vi "Microfone3.vi"() -> ()   [LabVIEW 2014]
uses:
  <vilib>/myRIO/Instrument Drivers/Onboard IO/AI/typedefs/AI Reference.ctl
  <vilib>/myRIO/Common/Instrument Driver Framework/Utilities/typedefs/myRIO Generic Hardware Reference.ctl
  <vilib>/myRIO/Common/Instrument Driver Framework/Utilities/typedefs/Hardware Version Enum.ctl
  <vilib>/myRIO/Common/Instrument Driver Framework/Utilities/typedefs/myRIO v1.0 Reference.ctl
  <vilib>/myRIO/Common/Instrument Driver Framework/Utilities/typedefs/Generic FPGA Reference.ctl
  <vilib>/myRIO/Common/Instrument Driver Framework/myRIO v1.0/AI/typedefs/AI Channels List.ctl
  <vilib>/myRIO/Common/Instrument Driver Framework/myRIO v1.0/AI/typedefs/AI Channels Enum.ctl
  <vilib>/myRIO/Common/Instrument Driver Framework/Utilities/typedefs/Analog Scaling Constants List.ctl
  <vilib>/myRIO/Common/Instrument Driver Framework/Utilities/typedefs/Analog Scaling Constants.ctl
  <vilib>/userdefined/High Color/nirio_resource_hc.ctl
  <vilib>/myRIO/Common/Instrument Driver Framework/Utilities/vis/Is FPGA Ref Available.vi
  <vilib>/myRIO/Common/Instrument Driver Framework/myRIO v1.0/AI/vis/myRIO v1.1 Open AI.vi
  <vilib>/myRIO/Instrument Drivers/Onboard IO/AI/vis/Read.vi
  <vilib>/myRIO/Common/Instrument Driver Framework/Utilities/vis/Validate Channels.vi
  <vilib>/myRIO/Common/Instrument Driver Framework/myRIO v1.0/AI/vis/myRIO v1.0 Reserve AI.vi
  <vilib>/myRIO/Common/Instrument Driver Framework/myRIO v1.0/AI/vis/myRIO v1.0 Build MUX Configuration AI.vi
  <vilib>/myRIO/Common/Instrument Driver Framework/myRIO v1.0/Resource Manager/vis/myRIO v1.0 Reserve Channel List.vi
  <vilib>/myRIO/Common/Instrument Driver Framework/myRIO v1.0/Resource Manager/vis/myRIO v1.0 Reserve Channel.vi
  <vilib>/myRIO/Common/Instrument Driver Framework/myRIO v1.0/Resource Manager/vis/myRIO v1.0 Unreserve Channel.vi
  <vilib>/myRIO/Common/Instrument Driver Framework/myRIO v1.0/Resource Manager/vis/myRIO v1.0 Build Mutex Name.vi
  <vilib>/Utility/VariantDataType/GetNumericInfo.vi
  <vilib>/Utility/error.llb/Error Cluster From Error Code.vi
  <vilib>/myRIO/Common/Instrument Driver Framework/myRIO v1.0/myRIO v1.1 Open.vi
  <vilib>/myRIO/Common/Instrument Driver Framework/myRIO v1.0/AI/vis/myRIO v1.0 Get Scaling Constants AI.vi
  <vilib>/myRIO/Common/Instrument Driver Framework/Utilities/vis/IO Manager.vi
  <vilib>/myRIO/Common/Instrument Driver Framework/Utilities/vis/Configuration Manager.vi
  <vilib>/myRIO/Common/Instrument Driver Framework/myRIO v1.0/myRIO v1.0 Close.vi
  <vilib>/myRIO/Common/Instrument Driver Framework/myRIO v1.0/AI/vis/myRIO v1.0 Read AI.vi
  <vilib>/measure/matone.llb/Extract Multiple Tone Information N Chan.vi
  <vilib>/express/express analysis/Spectral/Block/exnSpectralBlock spectral measurements RMS poly.vi
  <vilib>/express/express analysis/Spectral/Block/exnSpectralBlock spectral measurements RMS DDT.vi
  <vilib>/myRIO/Express VI/Onboard IO/AI/AI Express VI.xnode
  <vilib>/myRIO/Instrument Drivers/Onboard IO/AI/vis/myRIO AI Open.xnode
  <vilib>/express/express analysis/Spectral/XNode/ExpressSpectralMeasurementsBlockNode.xnode
  <vilib>/measure/NI_MAPro.lvlib
  <vilib>/gmath/NI_Gmath.lvlib
  <vilib>/myRIO/Instrument Drivers/Onboard IO/AI/AI.lvlib
panel:
  out "size(s) 2":i32
  out "size(s)":i32
  out "XY Graph":cluster{"xi used":dbl[], "yi":dbl[]}(graph)
  in  "Threshold":dbl=0.001 format="%#_6p"
  out "Primeira amplitude":dbl
  out "Primeira frequência":dbl
  out "multiple tone information":T1(array[cluster]) {"multiple tone information"."detected phase (deg)" format="%_6g"; "multiple tone information"."detected amplitude" format="%_6p"; "multiple tone information"."detected frequency" format="%_6p"}
  in  "Stop Button":bool
  out "Espectro de Amplitudes":dynamicdata(graph)
  out "Waveform Graph":dynamicdata(graph)
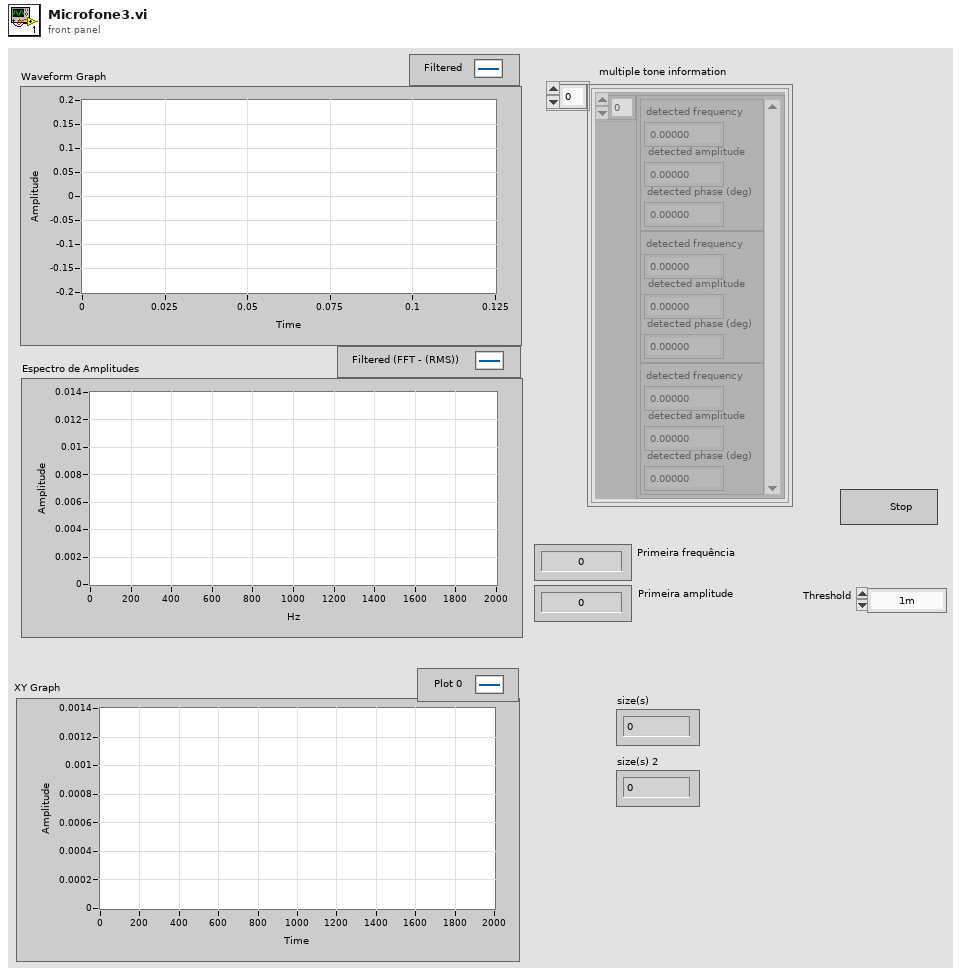
[diagram p1: front panel]
types:
  T1 = cluster{"multiple tone information":cluster{"detected frequency":dbl, "detected amplitude":dbl, "detected phase (deg)":dbl}[]}[]
  T2 = cluster{"averaging mode":u16, "weighting mode":u16, "number of averages":u32}
  T3 = cluster{"dB On (F)":bool, "unwrap phase (F)":bool, "convert to degree (F)":bool}
  T4 = typedef "AI.lvlib/AI Reference.ctl" = cluster{"myRIO Reference":T5, "AI Channels List":T9, "AI Scaling Constants List":T11}
  T5 = typedef "myRIO Generic Hardware Reference.ctl" = cluster{"myRIO Model":T6, "myRIO Hardware Reference":T7}
  T6 = typedef "Hardware Version Enum.ctl" = enum16{"Unknown", "myRIO-1900", "myRIO-1950"}
  T7 = typedef "myRIO v1.0 Reference.ctl" = cluster{"Generic FPGA Reference":T8, "Allow multiple opens":bool}
  T8 = typedef "Generic FPGA Reference.ctl" = refnum<k20>
  T9 = typedef "AI Channels List.ctl" = T10[]
  T10 = typedef "AI Channels Enum.ctl" = enum16{"Not Connected", "AudioIn/Left", "AudioIn/Right", "C/AI0", "C/AI1", "A/AI0", "A/AI1", "A/AI2", "A/AI3", "B/AI0", "B/AI1", "B/AI2", "B/AI3"}
  T11 = typedef "Analog Scaling Constants List.ctl" = T12[]
  T12 = typedef "Analog Scaling Constants.ctl" = cluster{"LSB Weight (Volts)":dbl, "Offset (Volts)":dbl, "Signed?":bool}
  T13 = typedef "nirio_resource_hc.ctl" = tag
  T14 = cluster{"multiple tone information":cluster{"detected frequency":dbl, "detected amplitude":dbl, "detected phase (deg)":dbl}[]}
  T15 = cluster{"detected frequency":dbl, "detected amplitude":dbl, "detected phase (deg)":dbl}[]
  T16 = cluster{"detected frequency":dbl, "detected amplitude":dbl, "detected phase (deg)":dbl}
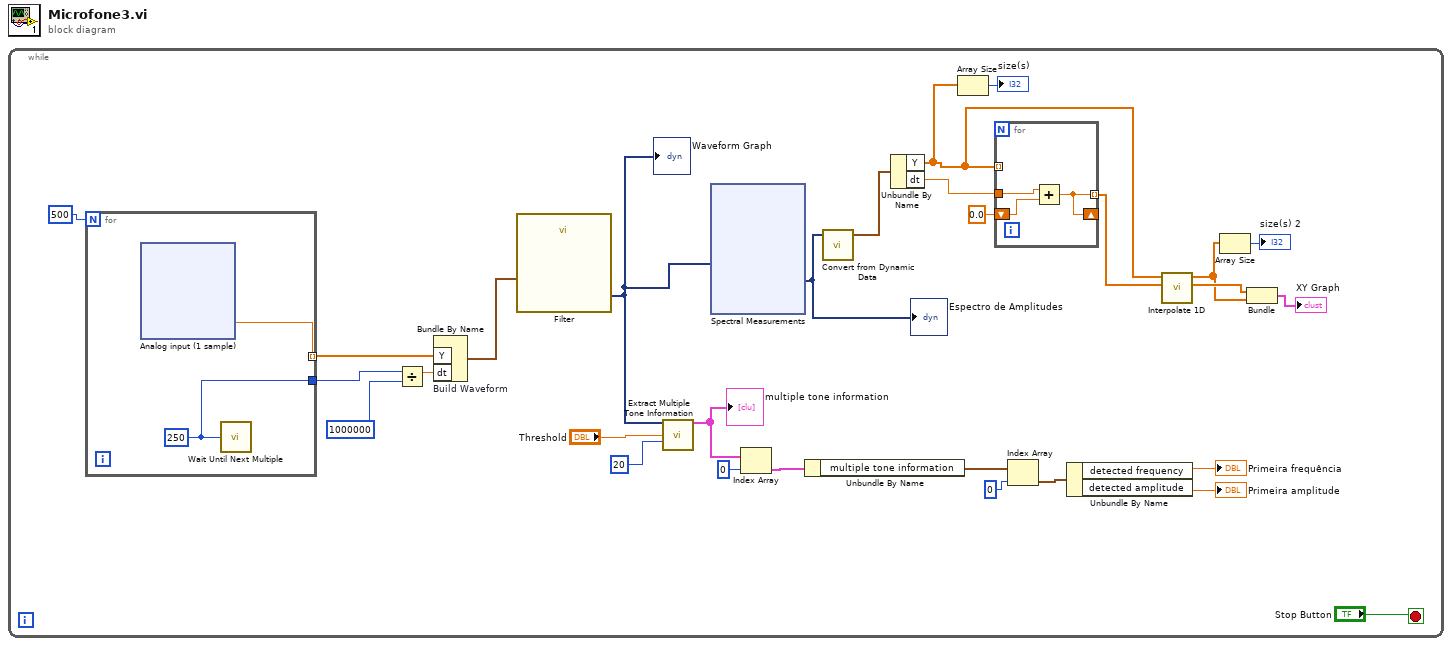
[diagram p0: block diagram]
diagram:
  n1 = while {
    stop <- "Stop Button" stop-if-true
    n2 = for {
      N: 500 -> [_]
      tunnel: [w44] -> w27 mode=indexing
      tunnel: [w43] -> w26
      w43 = u32 250 ("Count(uSec)")
      n3 = xnode "Analog input (1 sample)"() -> ("AudioIn/Left"=w44:dbl)  [unwired: 1 in, 1 out]
      n4 = call "Wait Until Next Multiple"("Count(uSec)"=w43) -> ()  [unwired: 1 out]
    }
    n5 = Divide(x=w26, y=u32 1000000) -> (x/y=w25:dbl)
    n6 = Bundle By Name "Build Waveform"("Y"=w27, "dt"=w25) -> (w23:waveform(dbl))  [unwired: 1 in]
    n7 = call "Filter"("Signal"=w23) -> ("Filtered Signal"=w22:dynamicdata)  [unwired: 9 in, 1 out]
    "Waveform Graph" <- w22
    n8 = call-poly <vilib>:"Extract Multiple Tone Information.vi"("time signals in"=w22, "threshold"="Threshold", "max num tones"=20) -> ("multiple tone information"=w21:T1)  [unwired: 10 in, 2 out]
    "multiple tone information" <- w21
    n9 = xnode "Spectral Measurements"("Signals"=w22) -> ("FFT - (RMS)"=w11:dynamicdata)  [unwired: 1 in, 2 out]
    "Espectro de Amplitudes" <- w11
    n10 = Index Array(array=w21, index=0) -> (element=w19:T14)
    n11 = Unbundle By Name(w19) -> ("multiple tone information"=w17:T15)
    n12 = call "Convert from Dynamic Data"("Dynamic Data Type"=w11) -> ("Waveform"=w10:waveform(dbl))  [unwired: 3 in]
    n13 = Unbundle By Name(w10) -> ("Y"=w4:dbl[], "dt"=w9:dbl)
    n14 = Array Size(array=w4) -> (size(s)=→"size(s)":i32)
    n15 = for {
      tunnel: w4 -> [_] mode=indexing
      tunnel: w9 -> [w32]
      tunnel: [w31] -> w7 mode=indexing
      shift-right: [w31] -> _
      shift-left: 0.0 -> [w30]
      n16 = Add(x=w32, y=w30) -> (x+y=w31:dbl)
    }
    n17 = Index Array(array=w17, index=0) -> (element=w16:T16)
    n18 = Unbundle By Name(w16) -> ("detected frequency"=→"Primeira frequência":dbl, "detected amplitude"=→"Primeira amplitude":dbl)
    n19 = call <vilib>:"Interpolate 1D.vi"("X"=w7, "Y"=w4) -> ("xi used"=w6:dbl[], "yi"=w1:dbl[])  [unwired: 7 in, 1 out]
    n20 = Array Size(array=w1) -> (size(s)=→"size(s) 2":i32)
    n21 = Bundle("xi used"=w6, "yi"=w1) -> (→"XY Graph":cluster{"xi used":dbl[], "yi":dbl[]})  [unwired: 1 in]
  }
